vi "Day 18 Puzzle 1.vi"(11 "Path":path) -> ()   [LabVIEW 2021]
uses:
  <vilib>/Utility/file.llb/Read Delimited Spreadsheet (string).vi
panel:
  out "subarray":string[](array[string])
  out "all rows":string[][](array[string])
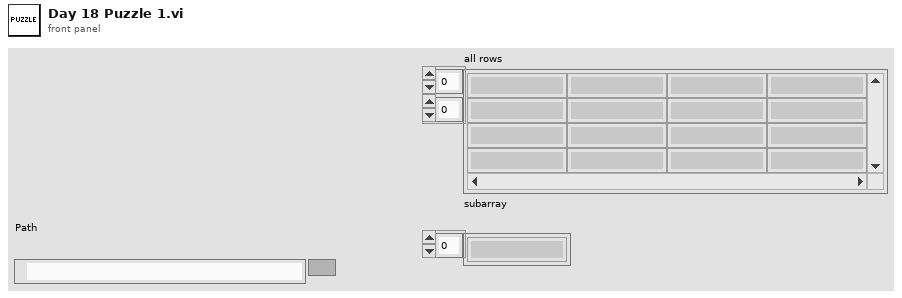
[diagram p1: front panel]
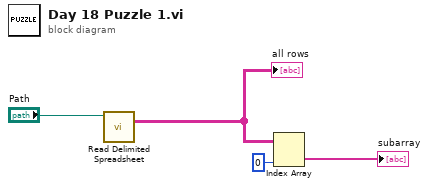
[diagram p0: block diagram]
diagram:
  n1 = call-poly <vilib>:"Read Delimited Spreadsheet.vi"("file path (dialog if empty)"="Path") -> ("all rows"=w3:string[][])  [unwired: 9 in, 5 out]
  "all rows" <- w3
  n2 = Index Array(array=w3, index (col)=0 ("disabled index (col)")) -> (element=→"subarray":string[])  [unwired: 1 in]
